vi "Climb Teleop.vi"(11 "Axes":dbl[](array[numeric])) -> ()   [LabVIEW 2020]
uses:
  Climb/Implementation/Climb Operations.ctl
  Axes.ctl
panel:
  in  "Operation":T1
  in  "Pivot Setpoint":dbl
  in  "Extension Setpoint":dbl
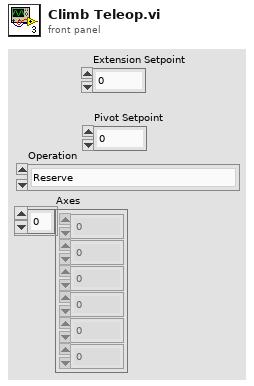
[diagram p1: front panel]
types:
  T1 = typedef "Climb Operations.ctl" = enum16{"Reserve", "Read Current", "Immediate", "Immediate Position", "Immediate Power"}
  T2 = typedef "Axes.ctl" = enum16{"LX", "LY", "LT", "RT", "RX", "RY"}
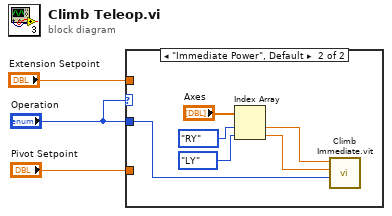
[diagram p0: block diagram]
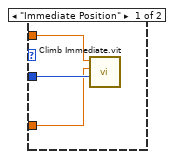
[diagram p2: hidden frame]
diagram:
  n1 = case shown="\"Immediate Power\", Default" "Operation" {
    tunnel: "Operation" -> [w6 w12]
    tunnel: "Extension Setpoint" -> [w5 _]
    tunnel: "Pivot Setpoint" -> [w4 _]
    frame "Immediate Position" {
      n2 = call "Climb Immediate.vit"("Operation"=w6, "Pivot"=w4, "Extension"=w5) -> ()  [unwired: 8 in, 1 out]
    }
    frame "Immediate Power", Default {
      n3 = Index Array(array="Axes", index #1=Axes."RY" ("Axes"), index #2=Axes."LY" ("Axes")) -> (element #1=w8:dbl, element #2=w7:dbl)
      n4 = call "Climb Immediate.vit"("Operation"=w12, "Pivot"=w7, "Extension"=w8) -> ()  [unwired: 8 in, 1 out]
    }
  }
